vi "uc480_SubVI_Example_PixelPeek.vi"(8 "Error In":errorcluster, 9 "Pos Y":i32, 10 "Pos X":i32, 11 ".NET (Reference)":refnum<k24>) -> (0 "Error Out":errorcluster, 1 "Blue":i32, 2 "Green":i32, 3 "Red":i32)   [LabVIEW 2011]
uses:
  C:/Program Files/Thorlabs/Scientific Imaging/DCx Camera Support/Develop/DotNet/uc480DotNet.dll
  Develop/DotNet/uc480DotNet.dll
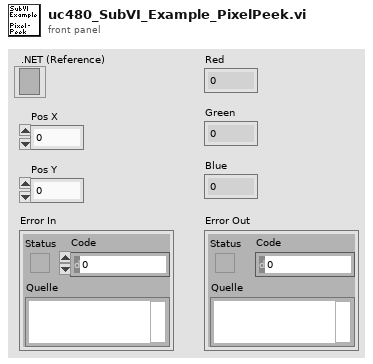
[diagram p1: front panel]
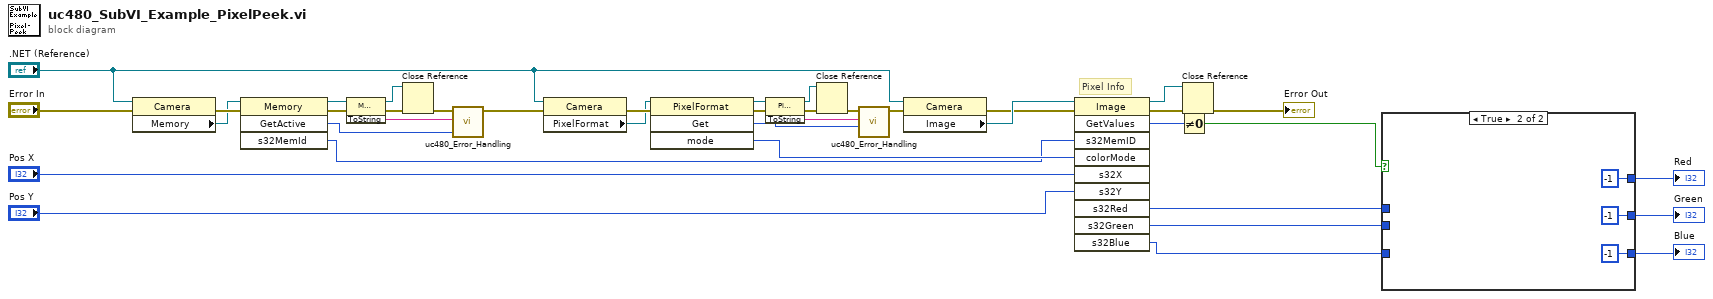
[diagram p0: block diagram]
diagram:
  # "Pixel Info"
  n1 = property class="Camera"(reference=".NET (Reference)", error in="Error In") -> (error out=w20:errorcluster, "Memory"=w19:refnum<k24>)  [unwired: 1 out]
  n2 = invoke class="Memory" method="GetActive"(reference=w19, error in=w20) -> (reference out=w25:refnum<k24>, error out=w24:errorcluster, "GetActive"=w23:i32, "s32MemId"=w21:i32)  [unwired: 2 in]
  n3 = invoke class="Memory" method="ToString"(reference=w25, error in=w24) -> (reference out=w7:refnum<k24>, error out=w9:errorcluster, "ToString"=w22:string)  [unwired: 1 in]
  n4 = Close Reference(reference=w7, error in (no error)=w9) -> (error out=w8:errorcluster)
  n5 = call "uc480_Error_Handling.vi"("Error Code"=w23, "Error String"=w22, "Error In"=w8) -> ("Error Out"=w38:errorcluster)  [unwired: 8 in]
  n6 = property on="Eigenschaftsknoten" class="Camera"(reference=".NET (Reference)", error in=w38) -> (error out=w29:errorcluster, "PixelFormat"=w28:refnum<k24>)  [unwired: 1 out]
  n7 = invoke class="PixelFormat" method="Get"(reference=w28, error in=w29) -> (reference out=w33:refnum<k24>, error out=w32:errorcluster, "Get"=w31:i32, "mode"=w35:i32)  [unwired: 2 in]
  n8 = invoke class="PixelFormat" method="ToString"(reference=w33, error in=w32) -> (reference out=w4:refnum<k24>, error out=w6:errorcluster, "ToString"=w30:string)  [unwired: 1 in]
  n9 = Close Reference(reference=w4, error in (no error)=w6) -> (error out=w5:errorcluster)
  n10 = call "uc480_Error_Handling.vi"("Error Code"=w31, "Error String"=w30, "Error In"=w5) -> ("Error Out"=w34:errorcluster)  [unwired: 8 in]
  n11 = property on="Eigenschaftsknoten" class="Camera"(reference=".NET (Reference)", error in=w34) -> (error out=w26:errorcluster, "Image"=w27:refnum<k24>)  [unwired: 1 out]
  n12 = invoke class="Image" method="GetValues"(reference=w27, error in=w26, "s32MemID"=w21, "colorMode"=w35, "s32X"="Pos X", "s32Y"="Pos Y") -> (reference out=w1:refnum<k24>, error out=w3:errorcluster, "GetValues"=w17:i32, "s32Red"=w15:i32, "s32Green"=w14:i32, "s32Blue"=w13:i32)  [unwired: 4 in, 4 out]
  n13 = Not Equal To 0?(x=w17) -> (x != 0?=w16:bool)
  n14 = Close Reference(reference=w1, error in (no error)=w3) -> (error out=→"Error Out":errorcluster)
  n15 = case shown="True" w16 {
    tunnel: w15 -> [w42 _]
    tunnel: w14 -> [w41 _]
    tunnel: w13 -> [w40 _]
    tunnel: [w42 -1 ("s32Red")] -> w12
    tunnel: [w41 -1 ("s32Green")] -> w11
    tunnel: [w40 -1 ("s32Blue")] -> w10
    frame False {
    }
    frame True {
    }
  }
  "Blue" <- w10
  "Green" <- w11
  "Red" <- w12
